vi "StateToStatusword.vi"(10 "StatusWord In":u16 format="%.0b", 11 "CurrentStatus":T1) -> (3 "StatusWord Out":u16 format="%08b")   [LabVIEW 2017, in "WordManipulationLibrary.lvlib"]
uses:
  WordManipulationLibrary.lvlib
  StateMachine.ctl
  Bit Manipulation.lvlib
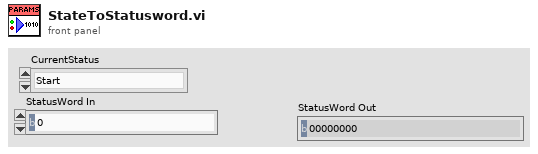
[diagram p1: front panel]
types:
  T1 = typedef "WordManipulationLibrary.lvlib/StateMachine.ctl" = enum16{"Start", "Not Ready to Switch On", "Switch On Disabled", "Ready to Switch On", "Switched On", "Operation enable", "Quick Stop Active", "Fault Reaction Active", "Fault"}
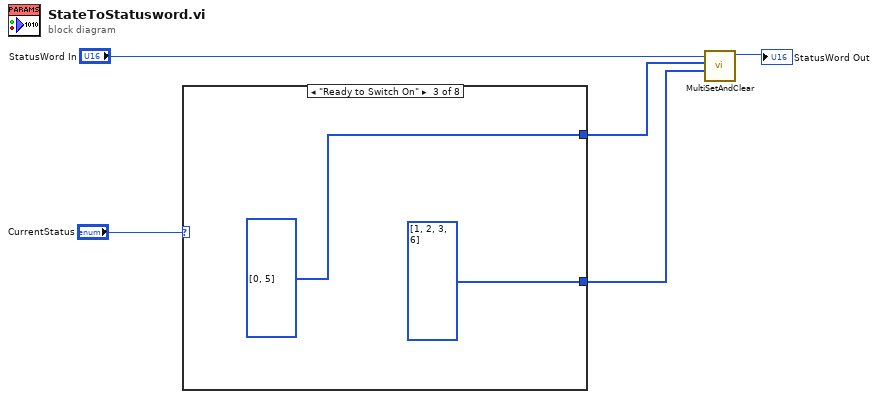
[diagram p0: block diagram]
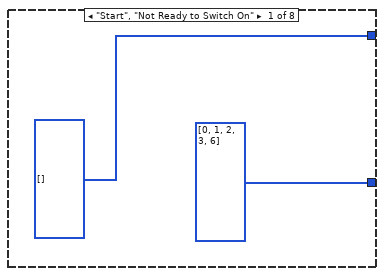
[diagram p2: hidden frame]
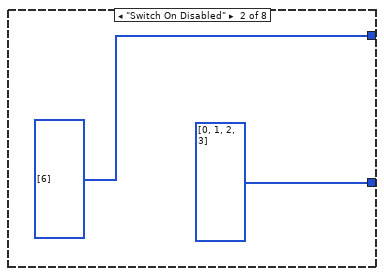
[diagram p3: hidden frame]
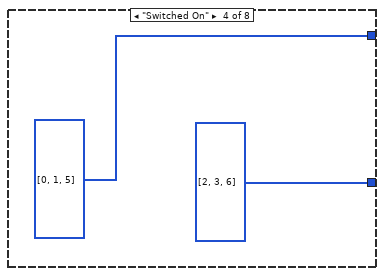
[diagram p4: hidden frame]
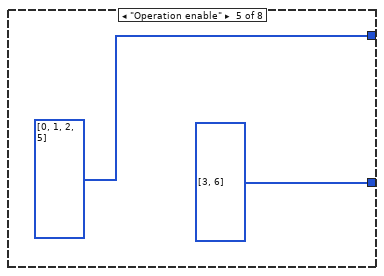
[diagram p5: hidden frame]
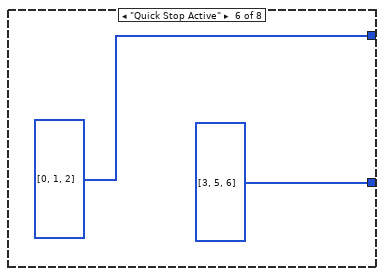
[diagram p6: hidden frame]
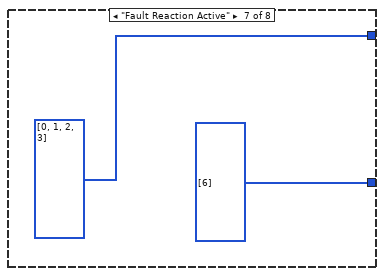
[diagram p7: hidden frame]
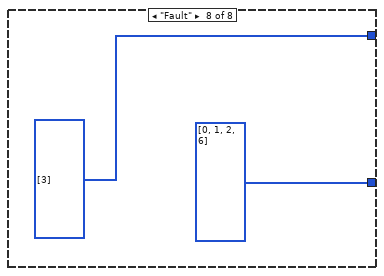
[diagram p8: hidden frame]
diagram:
  n1 = case shown="\"Ready to Switch On\"" "CurrentStatus" {
    tunnel: [u8[] [] u8[] [6] u8[] [0, 5] u8[] [0, 1, 5] u8[] [0, 1, 2, 5] u8[] [0, 1, 2] u8[] [0, 1, 2, 3] u8[] [3]] -> w2
    tunnel: [u8[] [0, 1, 2, 3, 6] u8[] [0, 1, 2, 3] u8[] [1, 2, 3, 6] u8[] [2, 3, 6] u8[] [3, 6] u8[] [3, 5, 6] u8[] [6] u8[] [0, 1, 2, 6]] -> w1
    frame "Start", "Not Ready to Switch On" {
    }
    frame "Switch On Disabled" {
    }
    frame "Ready to Switch On" {
    }
    frame "Switched On" {
    }
    frame "Operation enable" {
    }
    frame "Quick Stop Active" {
    }
    frame "Fault Reaction Active" {
    }
    frame "Fault" {
    }
  }
  n2 = call "MultiSetAndClear.vi"("Bits_To_Clear"=w1, "Bits_To_Set"=w2, "Data_in"="StatusWord In") -> ("Data_Out"=→"StatusWord Out":u16)  [unwired: 8 in]
